vi "find_fpwm.vi"(8 "Y":dbl[](array[numeric]), 10 "baseline":dbl=2000.0 format="%#_13g", 11 "X":dbl[](array[numeric])) -> (0 "falling":dbl, 1 "FPWM":dbl, 2 "rasing":dbl, 3 "center wavelength":dbl, 4 "center2":dbl)   [LabVIEW 2018]
uses:
  <vilib>/Analysis/NI_AALPro.lvlib
panel:
  out "XY图":cluster{"X":dbl[], "Best Gaussian Fit":dbl[]}[](graph)
  out "falling 10":dbl
  out "falling 90":dbl
  out "rasing 10":dbl
  out "rasing 90":dbl
  out "max":dbl
  out "后":dbl
  out "前":dbl
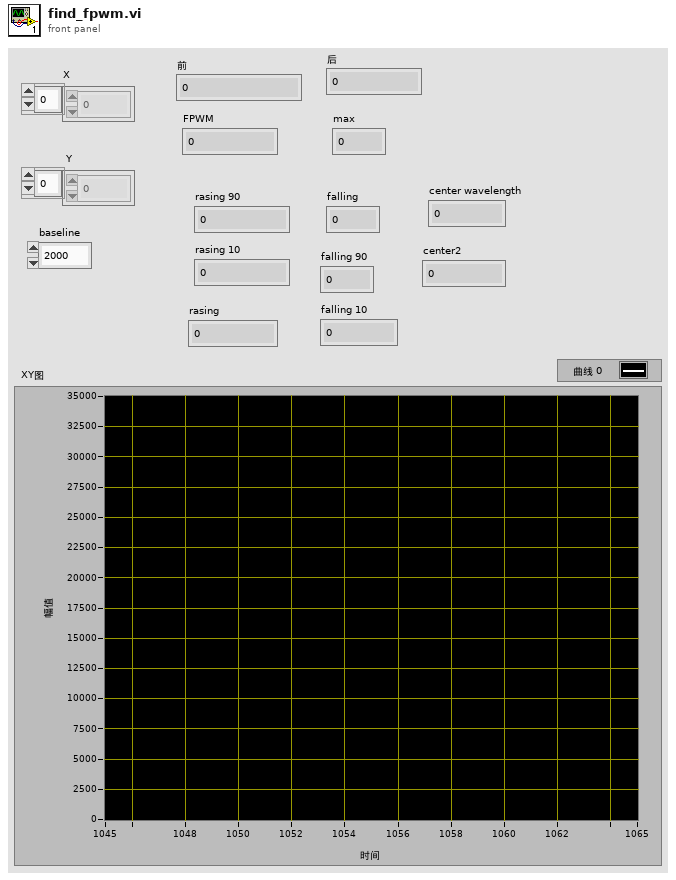
[diagram p1: front panel]
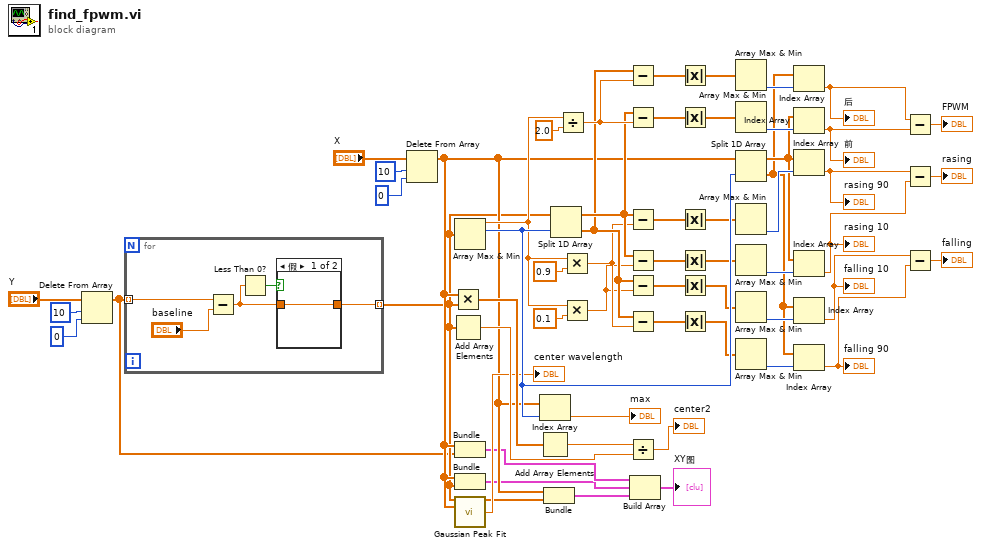
[diagram p0: block diagram]
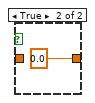
[diagram p2: hidden frame]
diagram:
  n1 = Delete From Array(array="Y", length=10 ("长度"), index=0 ("索引")) -> (array with subset deleted=w1:dbl[])  [unwired: 1 out]
  n2 = for {
    tunnel: w1 -> [w63] mode=indexing
    tunnel: [w64] -> w2 mode=indexing
    n3 = Subtract(x=w63, y="baseline") -> (x-y=w60:dbl)
    n4 = Less Than 0?(x=w60) -> (x < 0?=w61:bool)
    n5 = case shown="假" w61 {
      tunnel: [w65 0.0] -> w64
      tunnel: w60 -> [w65 _]
      frame False {
      }
      frame True {
      }
    }
  }
  n6 = Delete From Array(array="X", length=10 ("长度"), index=0 ("索引")) -> (array with subset deleted=w8:dbl[])  [unwired: 1 out]
  n7 = Multiply(x=w8, y=w2) -> (x*y=w14:dbl[])
  n8 = Add Array Elements(numeric array=w2) -> (sum=w12:dbl)
  n9 = Array Max & Min(array=w2) -> (max value=w39:dbl, max index (indices)=w50:i32)  [unwired: 2 out]
  n10 = Bundle("X"=w8, "Y"=w1) -> (w6:cluster{"X":dbl[], " Y":dbl[]})  [unwired: 1 in]
  n11 = Bundle("X"=w8, w2) -> (w5:cluster{"X":dbl[], dbl[]})  [unwired: 1 in]
  n12 = call <vilib>:"Gaussian Peak Fit.vi"("Y"=w2, "X"=w8) -> ("Best Gaussian Fit"=w7:dbl[], "center"=→"center wavelength":dbl)  [unwired: 7 in, 5 out]
  n13 = Index Array(array=w8, index=w50) -> (element=→"max":dbl)
  n14 = Add Array Elements(numeric array=w14) -> (sum=w13:dbl)
  n15 = Bundle("X"=w8, "Best Gaussian Fit"=w7) -> (w4:cluster{"X":dbl[], "Best Gaussian Fit":dbl[]})  [unwired: 1 in]
  n16 = Split 1D Array(array=w2, index=w50) -> (first subarray=w38:dbl[], second subarray=w21:dbl[])
  n17 = Divide(x=w39, y=2.0) -> (x/y=w56:dbl)
  n18 = Multiply(x=w39, y=0.9) -> (x*y=w20:dbl)
  n19 = Multiply(x=w39, y=0.1) -> (x*y=w19:dbl)
  n20 = Subtract(x=w21, y=w56) -> (x-y=w55:dbl[])
  n21 = Subtract(x=w38, y=w56) -> (x-y=w58:dbl[])
  n22 = Subtract(x=w38, y=w20) -> (x-y=w37:dbl[])
  n23 = Subtract(x=w38, y=w19) -> (x-y=w36:dbl[])
  n24 = Subtract(x=w21, y=w19) -> (x-y=w26:dbl[])
  n25 = Subtract(x=w21, y=w20) -> (x-y=w27:dbl[])
  n26 = Divide(x=w13, y=w12) -> (x/y=→"center2":dbl)
  n27 = Build Array(w6, w5, w4) -> (→"XY图":cluster{"X":dbl[], "Best Gaussian Fit":dbl[]}[])
  n28 = Absolute Value(x=w55) -> (abs(x)=w54:dbl[])
  n29 = Absolute Value(x=w58) -> (abs(x)=w57:dbl[])
  n30 = Absolute Value(x=w37) -> (abs(x)=w35:dbl[])
  n31 = Absolute Value(x=w36) -> (abs(x)=w34:dbl[])
  n32 = Absolute Value(x=w26) -> (abs(x)=w24:dbl[])
  n33 = Absolute Value(x=w27) -> (abs(x)=w25:dbl[])
  n34 = Array Max & Min(array=w54) -> (min index (indices)=w52:i32)  [unwired: 3 out]
  n35 = Array Max & Min(array=w57) -> (min index (indices)=w53:i32)  [unwired: 3 out]
  n36 = Split 1D Array(array=w8, index=w50) -> (first subarray=w31:dbl[], second subarray=w18:dbl[])
  n37 = Array Max & Min(array=w35) -> (min index (indices)=w33:i32)  [unwired: 3 out]
  n38 = Array Max & Min(array=w34) -> (min index (indices)=w32:i32)  [unwired: 3 out]
  n39 = Array Max & Min(array=w24) -> (min index (indices)=w22:i32)  [unwired: 3 out]
  n40 = Array Max & Min(array=w25) -> (min index (indices)=w23:i32)  [unwired: 3 out]
  n41 = Index Array(array=w18, index=w52) -> (element=w44:dbl)
  "后" <- w44
  n42 = Index Array(array=w31, index=w53) -> (element=w43:dbl)
  "前" <- w43
  n43 = Index Array(array=w31, index=w33) -> (element=w30:dbl)
  "rasing 90" <- w30
  n44 = Index Array(array=w31, index=w32) -> (element=w29:dbl)
  "rasing 10" <- w29
  n45 = Index Array(array=w18, index=w22) -> (element=w17:dbl)
  "falling 10" <- w17
  n46 = Index Array(array=w18, index=w23) -> (element=w16:dbl)
  "falling 90" <- w16
  n47 = Subtract(x=w44, y=w43) -> (x-y=→"FPWM":dbl)
  n48 = Subtract(x=w30, y=w29) -> (x-y=→"rasing":dbl)
  n49 = Subtract(x=w17, y=w16) -> (x-y=→"falling":dbl)
